vi "RSNRPZ Set Correction Frequency Step.vi"(8 "error in (no error)":errorcluster, 9 "Frequency Step (0.0)":dbl format="%^.3e", 10 "Channel (1)":i32=1, 11 "VISA session":refnum<visa-resource-name> caption="VISA resource name") -> (0 "error out":errorcluster, 3 "dup VISA session":refnum<visa-resource-name> caption="VISA resource name")   [LabVIEW 2010]
doc: "If the frequency step parameter is set to a value greater than 0.0 the sensor does a internal frequency increment if buffered mode is enabled\n\nDepending on the parameter \"frequency spacing\" the sensor adds this value to the current frequency or it multiplies this value with the current frequency.\n\nThis VI is used to do a simple scalar network nalysis. \nTo enable this automativally frequency stepping you have to configure CONTAV sensor mode, enable buffered measurements and set frequency stepping to a value greater than 0.\n\nRemote-control command(s):\nSENS:FREQ:STEP"
uses:
  rsnrpz_32.dll
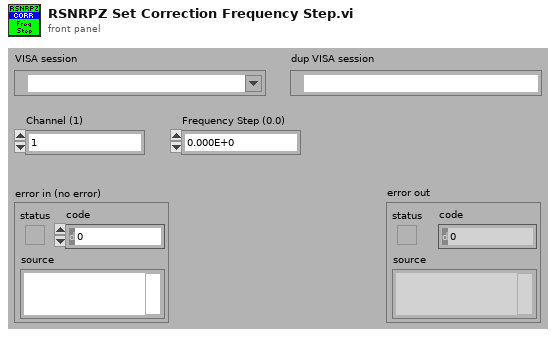
[diagram p1: front panel]
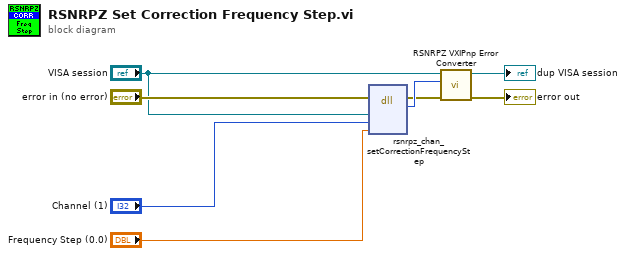
[diagram p0: block diagram]
diagram:
  n1 = dll-call lib="rsnrpz_32.dll" fn="rsnrpz_chan_setCorrectionFrequencyStep"(error in="error in (no error)", "Instrument Handle"="VISA session", "Channel"="Channel (1)", "Frequency Step"="Frequency Step (0.0)") -> (error out=w5:errorcluster, w6:i32)  [unwired: 5 in, 1 out]
  n2 = call <instrlib>:"RSNRPZ VXIPnp Error Converter.vi"("error in"=w5, "VXIPnp error code"=w6, "VISA session"="VISA session") -> ("error out"=→"error out":errorcluster, "dup VISA session"=→"dup VISA session":refnum<visa-resource-name>)  [unwired: 7 in]
